vi "Get MLJ Stage Enabled.vi"(8 "error in (no error)":errorcluster, 10 "Cluster in":T1, 11 "MLJ Reference In":refnum<k24>) -> (0 "error out":errorcluster, 1 "IsEnabled":bool, 2 "Cluster out":T1, 3 "MLJ Reference Out":refnum<k24>)   [LabVIEW 2018]
uses:
  Controls/Translation Stage Cluster.ctl
  General/Controls/Translation Stage Types.ctl
  C:/Project/SerialSectionOCT/SerialSectOCT/Labview Software/Thorlabs.MotionControl.Controls.dll
  Thorlabs.MotionControl.Controls.dll
  C:/Project/SerialSectionOCT/SerialSectOCT/Labview Software/Thorlabs.MotionControl.IntegratedStepperMotorsCLI.dll
  Thorlabs.MotionControl.IntegratedStepperMotorsCLI.dll
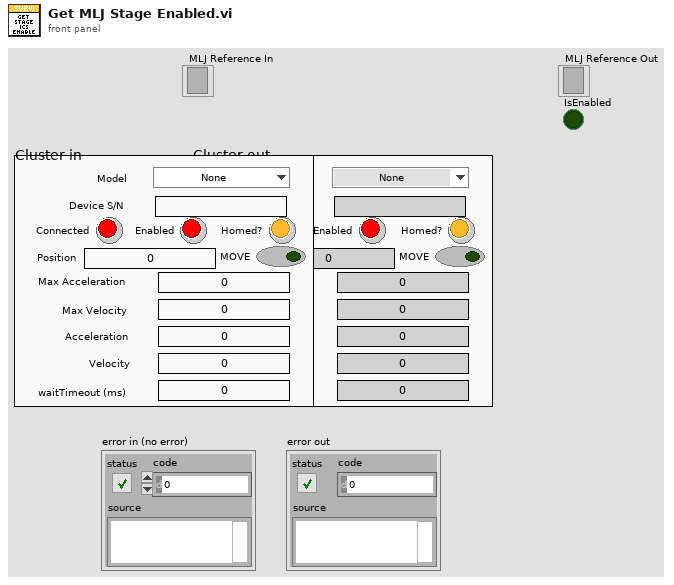
[diagram p1: front panel]
types:
  T1 = typedef "Translation Stage Cluster.ctl" = cluster{"Position":dbl, "Is.Enabled?":bool, "Is.Connected?":bool, "Device SN":string, "AccelerationMaximum":dbl, "VelocityMaximum":dbl, "Acceleration":dbl, "Velocity":dbl, "waitTimeout (ms)":i32, "Model":T2, "Is.Homed?":bool, "MOVE":bool}
  T2 = typedef "Translation Stage Types.ctl" = enum16{"None", "Thorlabs LTS", "Thorlabs MLJ"}
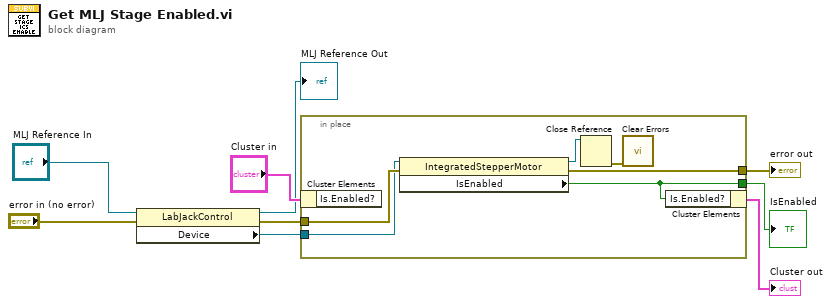
[diagram p0: block diagram]
diagram:
  n1 = property class="LabJackControl"(reference="MLJ Reference In", error in="error in (no error)") -> (reference out=→"MLJ Reference Out":refnum<k24>, error out=w4:errorcluster, "Device"=w1:refnum<k24>)
  n2 = in-place {
    in-place-border: w4 -> [w15]
    in-place-border: [w14] -> w7
    in-place-border: [w11] -> w6
    in-place-border: w1 -> [w10]
    n3 = in-place-cluster #1("Cluster in") -> ()  [unwired: 1 out]
    n4 = property class="IntegratedStepperMotor"(reference=w10, error in=w15) -> (reference out=w12:refnum<k24>, error out=w14:errorcluster, "IsEnabled"=w11:bool)
    n5 = Close Reference(reference=w12) -> (error out=w13:errorcluster)  [unwired: 1 in]
    n6 = call <vilib>:"Clear Errors.vi"("error in (no error)"=w13) -> ()  [unwired: 5 in, 2 out]
    n7 = in-place-cluster #1("Is.Enabled?"=w11) -> (→"Cluster out":T1)
  }
  "error out" <- w7
  "IsEnabled" <- w6
